vi "load_I_T_from_file.vi"() -> ()   [LabVIEW 2016]
uses:
  <vilib>/Utility/file.llb/Read Delimited Spreadsheet (DBL).vi
panel:
  in  "Proceed to Input Data":bool
  in  "# Nodes Per Stage":dbl[](array[numeric])
  in  "# Hidden Layers":dbl
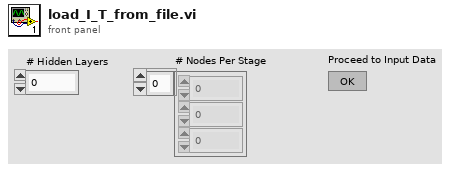
[diagram p1: front panel]
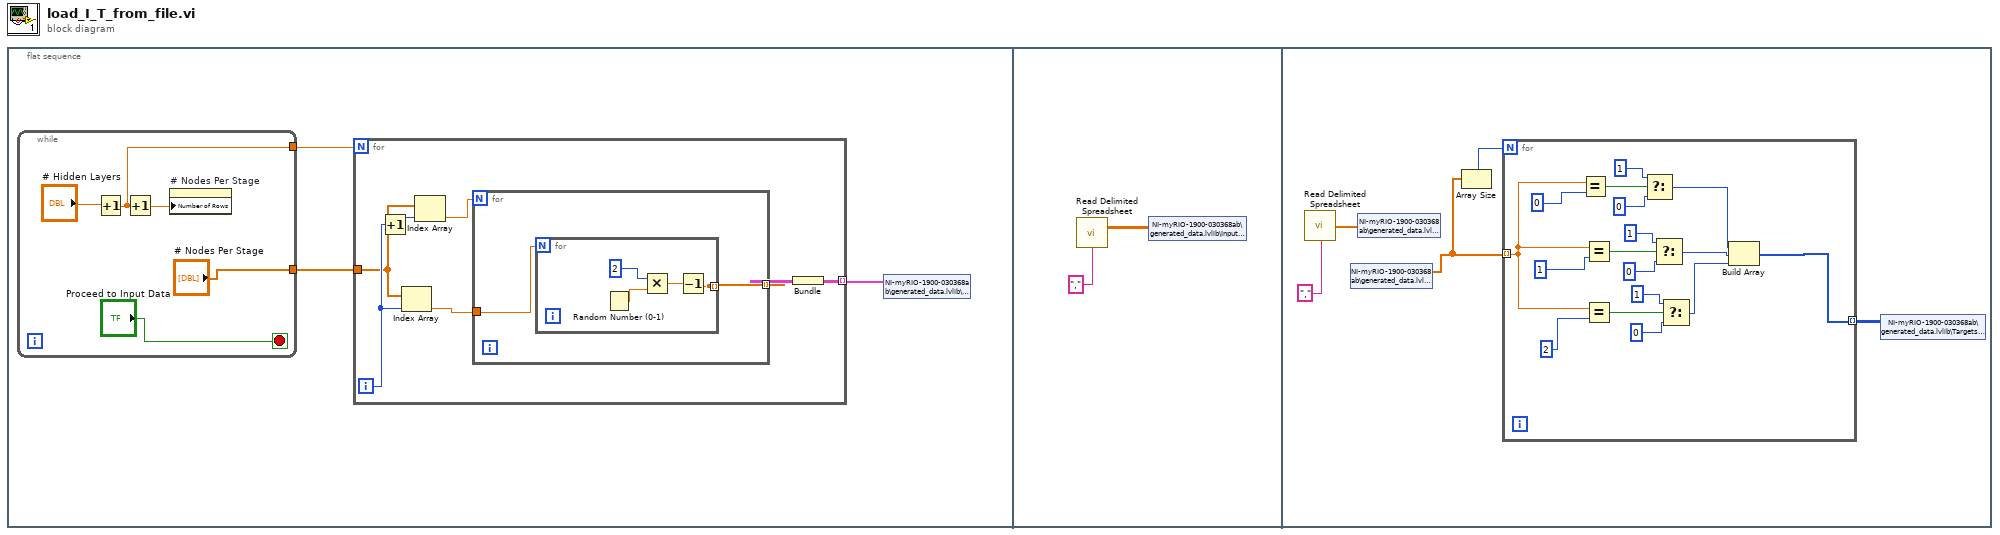
[diagram p0: block diagram]
diagram:
  n1 = flat-sequence {
    frame #0 {
      n2 = while {
        tunnel: [w5] -> w2
        tunnel: ["# Nodes Per Stage"] -> w1
        stop <- "Proceed to Input Data" stop-if-true
        n3 = Increment(x="# Hidden Layers") -> (x+1=w5:dbl)
        n4 = Increment(x=w5) -> (x+1=w8:dbl)
        n5 = property on="# Nodes Per Stage" class="Arr (strict)"("Number of Rows"=w8) -> ()  [unwired: 2 in, 2 out]
      }
      n6 = for {
        N: w2 -> [_]
        tunnel: [w14] -> w3 mode=indexing
        tunnel: w1 -> [w11]
        i -> [w13]
        n7 = Increment(x=w13) -> (x+1=w12:i32)
        n8 = Index Array(array=w11, index=w13) -> (element=w9:dbl)
        n9 = Index Array(array=w11, index=w12) -> (element=w10:dbl)
        n10 = for {
          N: w10 -> [_]
          tunnel: [w17] -> w15 mode=indexing
          tunnel: w9 -> [w16]
          n11 = for {
            N: w16 -> [_]
            tunnel: [w21] -> w17 mode=indexing
            n12 = Random Number (0-1)() -> (number: 0 to 1=w19:dbl)
            n13 = Multiply(x=2, y=w19) -> (x*y=w18:dbl)
            n14 = Decrement(x=w18) -> (x-1=w21:dbl)
          }
        }
        n15 = Bundle(w15) -> (w14:cluster{dbl[][]})  [unwired: 1 in]
      }
      n16 = shared-variable "NI-myRIO-1900-030368ab\\generated_data.lvlib\\Weights"(w3) -> ()  [unwired: 1 in, 1 out]
    }
    frame #1 {
      n17 = call-poly <vilib>:"Read Delimited Spreadsheet.vi"("delimiter (\\t)"=",") -> ("all rows"=w23:dbl[][])  [unwired: 9 in, 5 out]
      n18 = shared-variable "NI-myRIO-1900-030368ab\\generated_data.lvlib\\Input Data"(w23) -> ()  [unwired: 1 in, 1 out]
    }
    frame #2 {
      n19 = call-poly <vilib>:"Read Delimited Spreadsheet.vi"("delimiter (\\t)"=",") -> ("first row"=w28:dbl[])  [unwired: 9 in, 5 out]
      n20 = shared-variable "NI-myRIO-1900-030368ab\\generated_data.lvlib\\Targets"() -> (w24:dbl[])  [unwired: 1 in, 1 out]
      n21 = shared-variable "NI-myRIO-1900-030368ab\\generated_data.lvlib\\Targets"(w28) -> ()  [unwired: 1 in, 1 out]
      n22 = Array Size(array=w24) -> (size(s)=w25:i32)
      n23 = for {
        N: w25 -> [_]
        tunnel: w24 -> [w44] mode=indexing
        tunnel: [w29] -> w26 mode=indexing
        n24 = Equal?(x=w44, y=0) -> (x = y?=w41:bool)
        n25 = Equal?(x=w44, y=1) -> (x = y?=w33:bool)
        n26 = Equal?(x=w44, y=2) -> (x = y?=w34:bool)
        n27 = Select(t=1, s=w41, f=0) -> (s? t:f=w32:i32)
        n28 = Select(t=1, s=w33, f=0) -> (s? t:f=w31:i32)
        n29 = Select(t=1, s=w34, f=0) -> (s? t:f=w30:i32)
        n30 = Build Array(w32, w31, w30) -> (w29:i32[])
      }
      n31 = shared-variable "NI-myRIO-1900-030368ab\\generated_data.lvlib\\Targets_OH"(w26) -> ()  [unwired: 1 in, 1 out]
    }
  }
